vi "Handle Last Ack Core.vi"(4 "error in (no error)":errorcluster, 6 "Last Ack":refnum<class "Last Ack.lvclass">, 7 "TEC Controller in":refnum<class "TEC Controller.lvclass">) -> (0 "error out":errorcluster, 3 "TEC Controller out":refnum<class "TEC Controller.lvclass">)   [LabVIEW 2014, in "Humidifier Test Lib.lvlib" / "TEC Controller.lvclass"]
doc: "(<B>Filename</B>: Actor Framework.lvlib:Actor.lvclass:Handle Last Ack Core.vi)\n\nDefines how the caller actor responds to the Last Ack message from a nested actor. The Last Ack message is the final message a nested actor sends to its caller before it shuts down. The message contains information about the final state of the nested actor.\n\nBy default, this method does nothing except return any error the nested actor sent. A descendant class may override this method to define behavior."
uses:
  TEC Controller.lvclass
  <vilib>/ActorFramework/LastAck/Last Ack.lvclass
  TEC Controller.lvclass/TEC Controller.ctl
  <vilib>/ActorFramework/Actor/Actor.lvclass/Actor.ctl
  <vilib>/ActorFramework/Message Enqueuer/Message Enqueuer.lvclass/Message Enqueuer.ctl
  <vilib>/ActorFramework/Message Enqueuer/Init from Existing Queue.vi
  <vilib>/ActorFramework/Message Enqueuer/Enqueue.vi
  <vilib>/ActorFramework/Message Priority Queue/Priority Enqueue.vi
  <vilib>/ActorFramework/Message Enqueuer/Message Enqueuer.lvclass
  <vilib>/ActorFramework/Stop Msg/Stop Msg.lvclass
  <vilib>/ActorFramework/Actor/Actor.lvclass
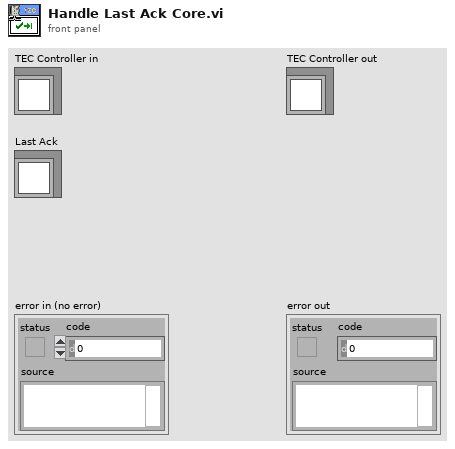
[diagram p1: front panel]
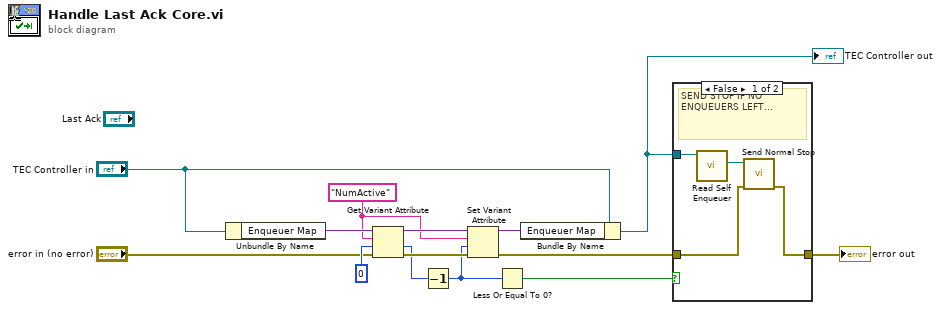
[diagram p0: block diagram]
diagram:
  w7 = "NumActive" ("name")
  n1 = Unbundle By Name("TEC Controller in") -> ("Enqueuer Map"=w14:variant)
  n2 = Get Variant Attribute(Variant=w14, name=w7, default value (empty Variant)=i16 0, error in="error in (no error)") -> (duplicate Variant=w13:variant, value=w5:i16, error out=w12:errorcluster)  [unwired: 1 out]
  n3 = Decrement(x=w5) -> (x-1=w10:i16)
  n4 = Set Variant Attribute(Variant=w13, name=w7, value=w10, error in=w12) -> (Variant out=w11:variant, error out=w8:errorcluster)  [unwired: 1 out]
  n5 = Less Or Equal To 0?(x=w10) -> (x <= 0?=w9:bool)
  n6 = Bundle By Name(cluster="TEC Controller in", "Enqueuer Map"=w11) -> (w4:refnum<class "TEC Controller.lvclass">)
  "TEC Controller out" <- w4
  n7 = case shown="False" w9 {
    tunnel: w4 -> [w17 _]
    tunnel: w8 -> [w16 w19]
    tunnel: [w15 w19] -> w1
    frame False {
      # "SEND STOP IF NO ENQUEUERS LEFT..."
      n8 = call <vilib>:"Read Self Enqueuer.vi"("Actor"=w17) -> ("Self Enqueuer"=w18:refnum<class "Message Enqueuer.lvclass">)  [unwired: 10 in]
      n9 = call <vilib>:"Send Normal Stop.vi"("error in (no error)"=w16, "Message Enqueuer"=w18) -> ("error out"=w15:errorcluster)  [unwired: 9 in]
    }
    frame True {
    }
  }
  "error out" <- w1
